vi "Refresh ESTTL Listbox.vi"(9 "Names":string[](array[string]), 10 "Setup":T1[](array[typedef]) caption="Differential I/O Setup" {"Skip Fire Index" max=7; "Angles"."Duration [s]" format="%#_3p"; "Frequency [Hz]" format="%#_3p"}, 11 "MulticolumnListbox in":refnum<vi>) -> ()   [LabVIEW 2016, in "DCM System Explorer.lvlib"]
uses:
  DCM System Explorer.lvlib
  <vilib>/Powertrain Controls/Device Drivers/DCM/ESTTL/RT/Setup.ctl
  <vilib>/Powertrain Controls/Device Drivers/DCM/ESTTL/FPGA/Mode.ctl
  <vilib>/Powertrain Controls/Device Drivers/DCM/ESTTL/RT/Angle Control.ctl
  <vilib>/Powertrain Controls/Device Drivers/DCM/ESTTL/RT/DCM - RT - ESTTL.lvlib
  <vilib>/Powertrain Controls/Device Drivers/DCM/ESTTL/FPGA/DCM - FPGA - ESTTL.lvlib
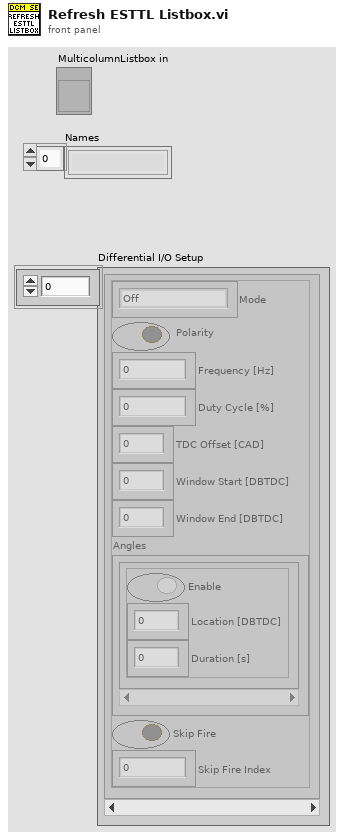
[diagram p1: front panel]
types:
  T1 = typedef "DCM - RT - ESTTL.lvlib/Setup.ctl" = cluster{"Mode":T2, "Polarity":bool, "Frequency [Hz]":sgl, "Duty Cycle [%]":sgl, "TDC Offset [CAD]":sgl, "Window Start [DBTDC]":sgl, "Window End [DBTDC]":sgl, "Angles":T3[], "Skip Fire":bool, "Skip Fire Index":u8}
  T2 = typedef "DCM - FPGA - ESTTL.lvlib/Mode.ctl" = enum8{"Off", "Pulse Width Modulation", "Engine Position Tracking"}
  T3 = typedef "DCM - RT - ESTTL.lvlib/Angle Control.ctl" = cluster{"Enable":bool, "Location [DBTDC]":sgl, "Duration [s]":sgl}
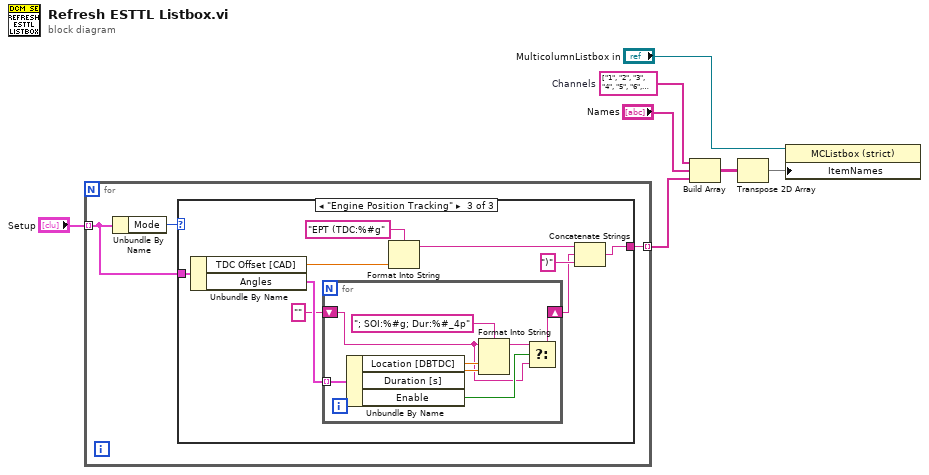
[diagram p0: block diagram]
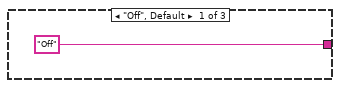
[diagram p2: hidden frame]
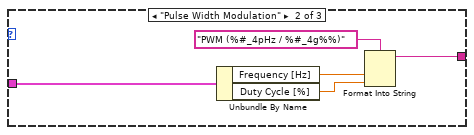
[diagram p3: hidden frame]
diagram:
  w5 = string[] ["1", "2", "3", "4", "5", "6", "7", "8", "9", "10", "11", "12", "13", "14", "15", "16"]  # Channels
  n1 = for {
    tunnel: "Setup" -> [w9] mode=indexing
    tunnel: [w8] -> w2 mode=indexing
    n2 = Unbundle By Name(w9) -> ("Mode"=w10:T2)
    n3 = case shown="\"Engine Position Tracking\"" w10 {
      tunnel: w9 -> [_ w16 w24]
      tunnel: ["Off" w12 w20] -> w8
      frame "Off", Default {
      }
      frame "Pulse Width Modulation" {
        n4 = Unbundle By Name(w16) -> ("Frequency [Hz]"=w14:sgl, "Duty Cycle [%]"=w13:sgl)
        n5 = Format Into String(format string="PWM (%#_4pHz / %#_4g%%)", w14, w13) -> (resulting string=w12:string)  [unwired: 2 in, 1 out]
      }
      frame "Engine Position Tracking" {
        n6 = Unbundle By Name(w24) -> ("TDC Offset [CAD]"=w23:sgl, "Angles"=w22:T3[])
        n7 = for {
          tunnel: w22 -> [w31] mode=indexing
          shift-right: [w27] -> w18
          shift-left: "" -> [w26]
          n8 = Unbundle By Name(w31) -> ("Location [DBTDC]"=w32:sgl, "Duration [s]"=w30:sgl, "Enable"=w29:bool)
          n9 = Format Into String(format string="; SOI:%#g; Dur:%#_4p", initial string=w26, w32, w30) -> (resulting string=w28:string)  [unwired: 1 in, 1 out]
          n10 = Select(t=w28, s=w29, f=w26) -> (s? t:f=w27:string)
        }
        n11 = Format Into String(format string="EPT (TDC:%#g", w23) -> (resulting string=w21:string)  [unwired: 2 in, 1 out]
        n12 = Concatenate Strings(w21, w18, ")" ("string")) -> (w20:string)
      }
    }
  }
  n13 = Build Array(w5, "Names", w2) -> (w7:string[][])
  n14 = Transpose 2D Array(2D array=w7) -> (transposed array=w4:string[][])
  n15 = property on="Property Node" class="MCListbox (strict)"(reference="MulticolumnListbox in", "ItemNames"=w4) -> ()  [unwired: 1 in, 2 out]
